vi "DiffDriveTrainSim_Pack_Simulation_Params.vi"(5 "X Pos Meas Std Dev M":dbl, 6 "Right Pos Meas Std Dev M":dbl, 7 "Y Pos Meas Std Dev M":dbl, 8 "Left Pos Meas Std Dev M":dbl, 9 "Right Vel Meas Std Dev M/S":dbl, 10 "Left Vel Meas Std Dev M/S":dbl, 11 "Heading Meas Std Dev Rad":dbl) -> (3 "DiffDriveSim_Simulation _Params":T1)   [LabVIEW 2019, in "Trajectory_Library.lvlib"]
uses:
  Trajectory_Library.lvlib
  TypeDef/DIFF_DRIVE_SIM_SIMULATION_PARAMS.ctl
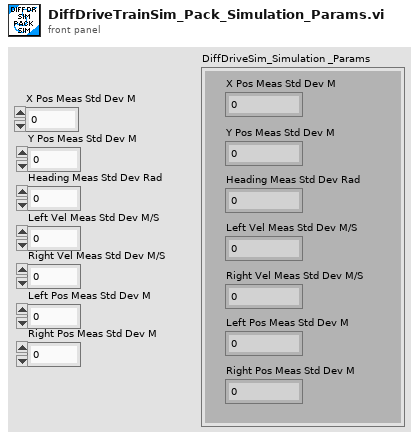
[diagram p1: front panel]
types:
  T1 = typedef "Trajectory_Library.lvlib/DIFF_DRIVE_SIM_SIMULATION_PARAMS.ctl" = cluster{"X Pos Meas Std Dev M":dbl, "Y Pos Meas Std Dev M":dbl, "Heading Meas Std Dev Rad":dbl, "Left Vel Meas Std Dev M/S":dbl, "Right Vel Meas Std Dev M/S":dbl, "Left Pos Meas Std Dev M":dbl, "Right Pos Meas Std Dev M":dbl}
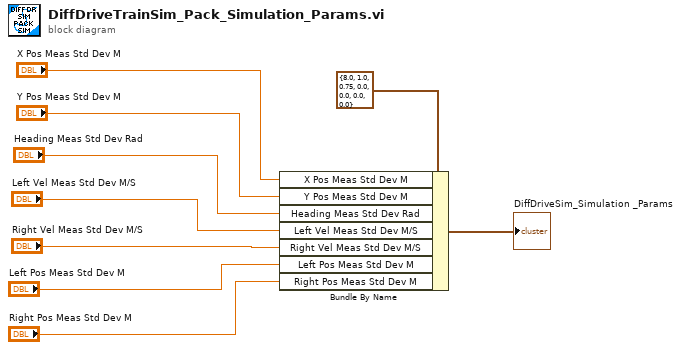
[diagram p0: block diagram]
diagram:
  n1 = Bundle By Name(cluster=T1 {"X Pos Meas Std Dev M"=8.0, "Y Pos Meas Std Dev M"=1.0, "Heading Meas Std Dev Rad"=0.75, "Left Vel Meas Std Dev M/S"=0.0, "Right Vel Meas Std Dev M/S"=0.0, "Left Pos Meas Std Dev M"=0.0, "Right Pos Meas Std Dev M"=0.0} ("SngJntArmSim_Simulation _Params"), "X Pos Meas Std Dev M"="X Pos Meas Std Dev M", "Y Pos Meas Std Dev M"="Y Pos Meas Std Dev M", "Heading Meas Std Dev Rad"="Heading Meas Std Dev Rad", "Left Vel Meas Std Dev M/S"="Left Vel Meas Std Dev M/S", "Right Vel Meas Std Dev M/S"="Right Vel Meas Std Dev M/S", "Left Pos Meas Std Dev M"="Left Pos Meas Std Dev M", "Right Pos Meas Std Dev M"="Right Pos Meas Std Dev M") -> (→"DiffDriveSim_Simulation _Params":T1)
